vi "ino.vi"() -> ()   [LabVIEW 2023]
uses:
  <vilib>/Instr/_visa.llb/VISA Configure Serial Port (Instr).vi
panel:
  in  "Stop":bool
  in  "write buffer":string
  in  "VISA resource name":refnum<visa-resource-name>
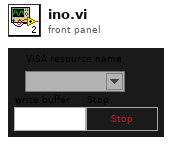
[diagram p1: front panel]
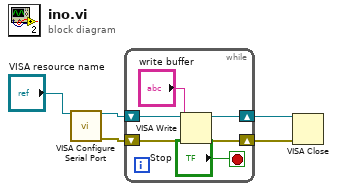
[diagram p0: block diagram]
diagram:
  n1 = call-poly "VISA Configure Serial Port"("VISA resource name"="VISA resource name") -> ("VISA resource name out"=w4:refnum<visa-resource-name>, "error out"=w3:errorcluster)  [unwired: 13 in]
  n2 = while {
    shift-right: [w9] -> w2
    shift-left: w4 -> [w11]
    shift-right: [w8] -> w1
    shift-left: w3 -> [w10]
    stop <- "Stop" stop-if-true
    n3 = VISA Write(VISA resource name=w11, write buffer="write buffer", error in (no error)=w10) -> (VISA resource name out=w9:refnum<visa-resource-name>, error out=w8:errorcluster)  [unwired: 1 out]
  }
  n4 = VISA Close(VISA resource name=w2, error in (no error)=w1) -> ()  [unwired: 1 out]
